vi "camera get one frame-subvi.vi"(2 "error in":errorcluster, 3 "New Image":T1) -> (0 "error out":errorcluster, 1 "Image Out":T1)   [LabVIEW 2014]
uses:
  <vilib>/vision/Image Controls.llb/IMAQ Image.ctl
  Initilize Globals.vi
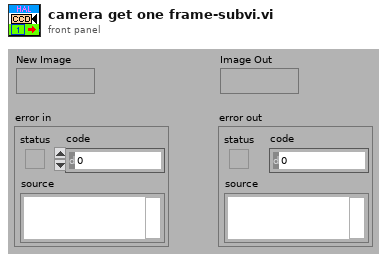
[diagram p1: front panel]
types:
  T1 = typedef "IMAQ Image.ctl" = refnum<image>
  T2 = cluster{"H Bin":dbl, "V Bin":dbl, "Left":dbl, "Right":dbl, "Top":dbl, "Bottom":dbl}
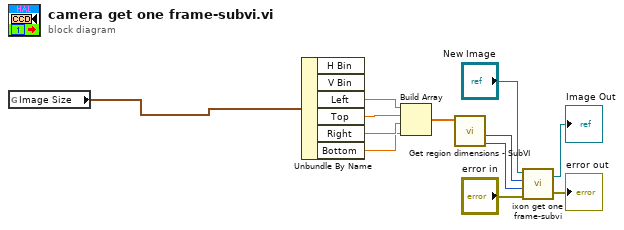
[diagram p0: block diagram]
diagram:
  n1 = global read "Initilize Globals.vi" "Image Size"() -> (w1:T2)
  n2 = Unbundle By Name(w1) -> ("Left"=w11:dbl, "Top"=w10:dbl, "Right"=w9:dbl, "Bottom"=w8:dbl)  [unwired: 2 out]
  n3 = Build Array(w11, w10, w9, w8) -> (w12:dbl[])
  n4 = call "Get region dimensions - SubVI.vi"("x1y1x2y2"=w12) -> ("y size"=w3:u16, "x size"=w4:u16)  [unwired: 7 in, 2 out]
  n5 = call "ixon get one frame-subvi.vi"("error in"="error in", "Image Height"=w3, "Image Width"=w4, "Image In"="New Image") -> ("error out"=→"error out":errorcluster, "Image Out"=→"Image Out":T1)  [unwired: 2 in]
